vi "MAIN_csv_to_csv_AUTO.vi"() -> ()   [LabVIEW 2017]
panel:
  out "Numeric":i32
  in  "frequency range":T1={"low band"=enum."20 Hz", "high band"=enum."20000 Hz"}
  in  "Canal":string[](array[string])=["cDAQ1Mod1_ai0"]
  in  "Largo de ventada \ntemporal en N samples":dbl=44100.0
  out "tdms":i32
  out "All Files in Dir":path[](array[path])
  in  "Referencias de TDMSs":path=path "D:/Registros_de_rodadura/Alcobendas02/TDMS&GPX"
  in  "Archivos de \nfeatures (.csv)":path=path "D:/Registros_de_rodadura/Alcobendas02/Feats_out"
  out "last\nconcatenated \nstring":string
  out "csvs de referencia)":i32
  out "filenames":string[](array[string])
  in  "Archivos de\nreferencias (.csv)":path=path "D:/Registros_de_rodadura/Alcobendas02/00_total_reff"
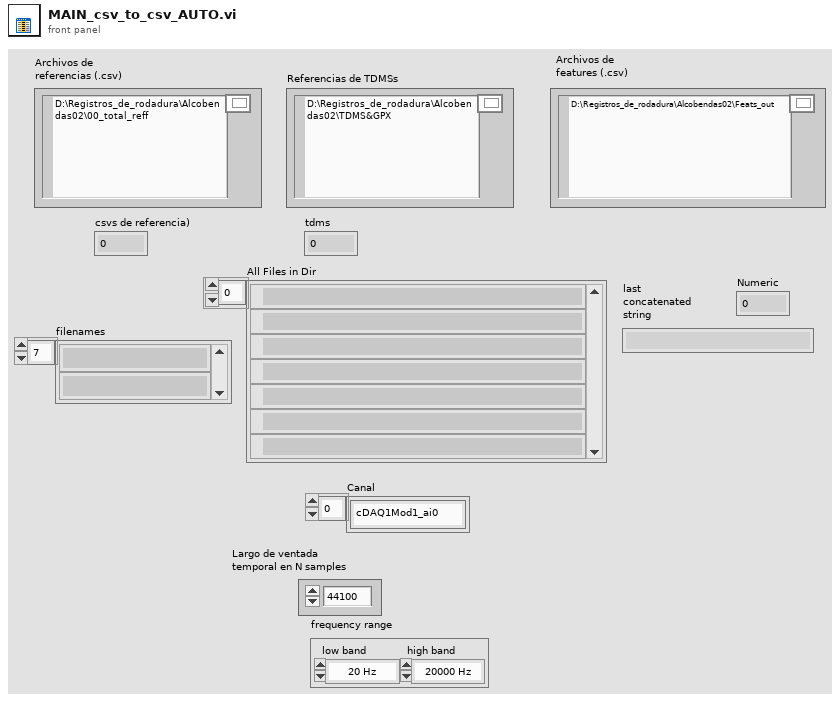
[diagram p1: front panel]
types:
  T1 = cluster{"low band":enum16{"20 Hz", "25 Hz", "31.5 Hz", "40 Hz", "50 Hz", "63 Hz", "80 Hz", "100 Hz", "125 Hz", "160 Hz", "200 Hz", "250 Hz", "315 Hz", "400 Hz", "500 Hz", "630 Hz", "800 Hz", "1000 Hz", "1250 Hz", "1600 Hz", "2000 Hz", "2500 Hz", "3150 Hz", "4000 Hz", "5000 Hz", "6300 Hz", "8000 Hz", "10000 Hz", "12500 Hz", "16000 Hz", "20000 Hz"}, "high band":enum16{"20 Hz", "25 Hz", "31.5 Hz", "40 Hz", "50 Hz", "63 Hz", "80 Hz", "100 Hz", "125 Hz", "160 Hz", "200 Hz", "250 Hz", "315 Hz", "400 Hz", "500 Hz", "630 Hz", "800 Hz", "1000 Hz", "1250 Hz", "1600 Hz", "2000 Hz", "2500 Hz", "3150 Hz", "4000 Hz", "5000 Hz", "6300 Hz", "8000 Hz", "10000 Hz", "12500 Hz", "16000 Hz", "20000 Hz"}}
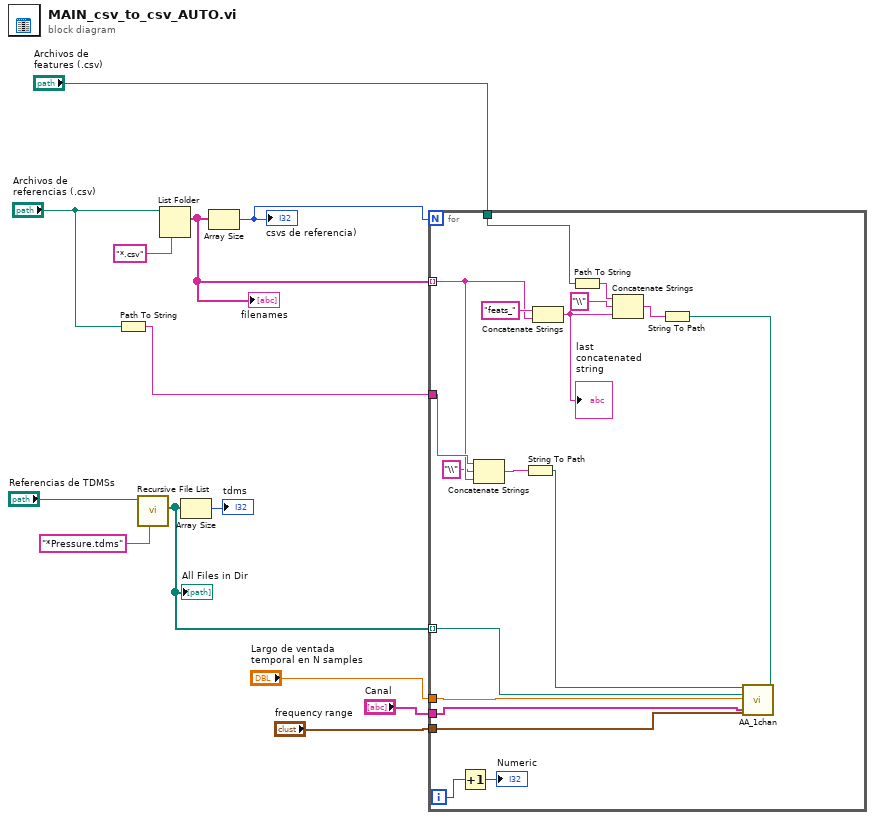
[diagram p0: block diagram]
diagram:
  n1 = Path To String(path="Archivos de\nreferencias (.csv)") -> (string=w5:string)
  n2 = call <vilib>:"Recursive File List.vi"("pattern"="*Pressure.tdms", "Folder Path"="Referencias de TDMSs") -> ("All Files in Dir"=w8:path[])  [unwired: 5 in, 4 out]
  "All Files in Dir" <- w8
  n3 = List Folder(path="Archivos de\nreferencias (.csv)", pattern="*.csv") -> (filenames=w7:string[])  [unwired: 2 in, 3 out]
  "filenames" <- w7
  n4 = Array Size(array=w8) -> (size(s)=→"tdms":i32)
  n5 = Array Size(array=w7) -> (size(s)=w1:i32)
  "csvs de referencia)" <- w1
  n6 = for {
    N: w1 -> [_]
    tunnel: w7 -> [w24] mode=indexing
    tunnel: "Archivos de \nfeatures (.csv)" -> [w22]
    tunnel: w8 -> [w20] mode=indexing
    tunnel: w5 -> [w26]
    tunnel: "Largo de ventada \ntemporal en N samples" -> [w19]
    tunnel: "Canal" -> [w18]
    tunnel: "frequency range" -> [w17]
    i -> [w16]
    n7 = Increment(x=w16) -> (x+1=→"Numeric":i32)
    n8 = Concatenate Strings(w26, "\\" ("string"), w24) -> (w25:string)
    n9 = String To Path(string=w25) -> (path=w21:path)
    n10 = Concatenate Strings("feats_", w24) -> (w29:string)
    "last\nconcatenated \nstring" <- w29
    n11 = Path To String(path=w22) -> (string=w30:string)
    n12 = Concatenate Strings(w30, "\\" ("string"), w29) -> (w27:string)
    n13 = String To Path(string=w27) -> (path=w14:path)
    n14 = call "AA_1chan.vi"("Archivo de\nreferencias (.csv)"=w21, "FEATS"=w14, "ARCHIVO\nTDMS"=w20, "Largo de ventada temporal en N samples"=w19, "Canal"=w18, "frequency range"=w17) -> ()  [unwired: 9 in, 1 out]
  }
